vi "Int64Array Destroy.vi"(8 "error in (no error)":errorcluster, 11 "Int64Array DVR in":refnum<data-value>) -> (0 "error out":errorcluster)   [LabVIEW 2015, in "MDSplus.lvlib"]
uses:
  <vilib>/MDSplus/Library/MDSplus.lvlib
  <vilib>/MDSplus/Classes/Data_Class/Array_Class/Int64Array_Class/Int64Array.lvclass
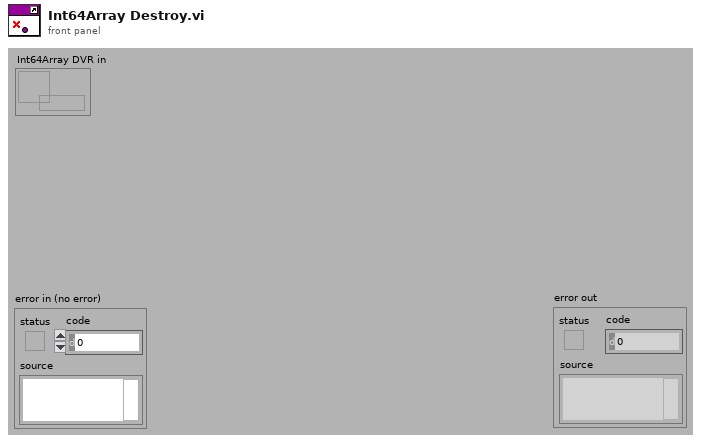
[diagram p1: front panel]
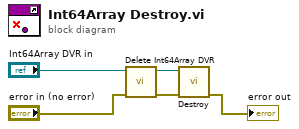
[diagram p0: block diagram]
diagram:
  n1 = call <vilib>:"Delete Int64Array DVR.vi"("error in (no error)"="error in (no error)", "Int64Array DVR in"="Int64Array DVR in") -> ("error out"=w2:errorcluster, "Int64Array out"=w3:refnum<class "Int64Array.lvclass">)  [unwired: 8 in]
  n2 = call-dynamic "Destroy.vi"("error in (no error)"=w2, "Int64Array in"=w3) -> ("error out"=→"error out":errorcluster)  [unwired: 9 in]
